vi "InitPCCamera.vi"(0 "index":i32) -> (1 "error out":errorcluster, 2 "cameraReference":i64, 3 "ret":i32)   [LabVIEW 2022 SP3]
uses:
  <vilib>/addons/RoboLab/ImageProcessing/WindowsDriver/LVDS.dll
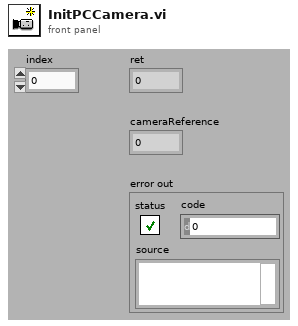
[diagram p1: front panel]
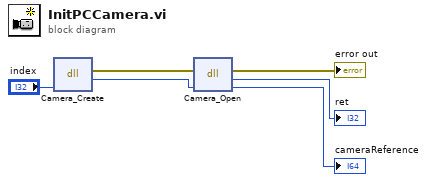
[diagram p0: block diagram]
diagram:
  n1 = dll-call lib="C:/Program Files (x86)/National Instruments/LabVIEW 2022/vi.lib/addons/RoboLab/ImageProcessing/WindowsDriver/LVDS.dll" fn="Camera_Create"("index"="index") -> (error out=w1:errorcluster, "cameraReference"=w2:i64)  [unwired: 4 in, 1 out]
  n2 = dll-call lib="C:/Program Files (x86)/National Instruments/LabVIEW 2022/vi.lib/addons/RoboLab/ImageProcessing/WindowsDriver/LVDS.dll" fn="Camera_Open"(error in=w1, "cameraReference"=w2) -> (error out=→"error out":errorcluster, "ret"=→"ret":i32, "cameraReference"=→"cameraReference":i64)  [unwired: 2 in, 1 out]
